vi "数值运算讲解.vi"() -> ()   [LabVIEW 2018]
uses:
  <vilib>/express/express arith-compare/Formula/XNode/ExpressFormulaBlockNode.xnode
panel:
  out "结果 2":dbl
  in  "X2":dbl
  in  "a 2":dbl
  out "y1":dbl
  in  "x":dbl
  out "数值 2":dbl
  in  "数值":dbl
  out "y":dbl
  in  "b":dbl
  in  "a":dbl
  out "结果":dbl
  in  "值 3":dbl
  in  "值 2":dbl
  in  "值":dbl
  # "y=2*a+b^2+5"
  # "y=x^2+3"
  # "y=a^2+x1^3"
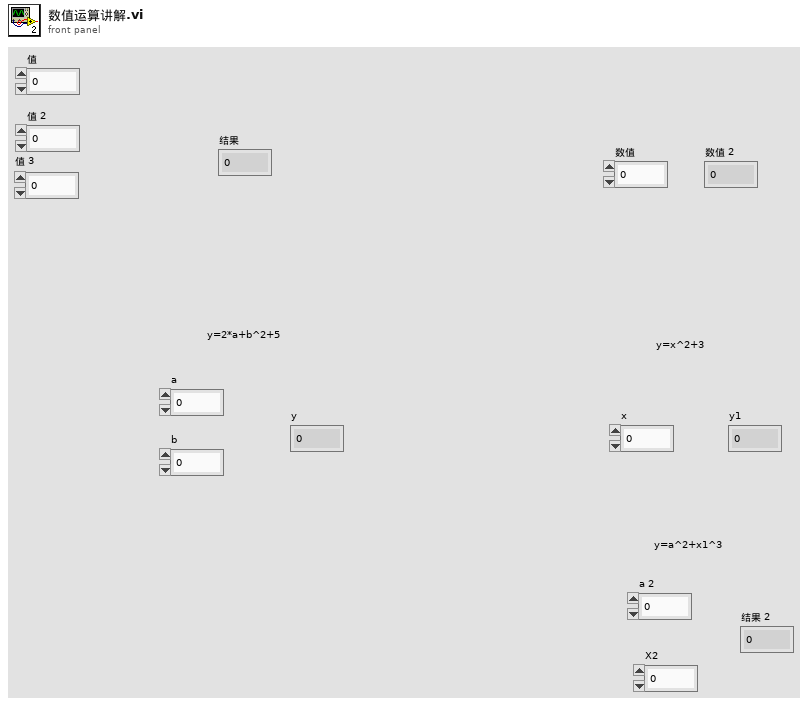
[diagram p1: front panel]
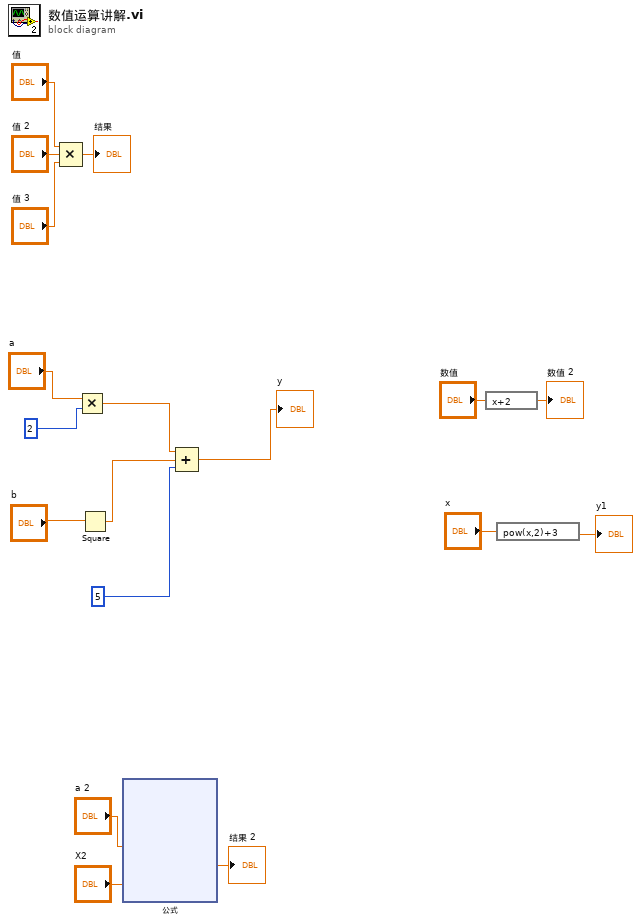
[diagram p0: block diagram]
diagram:
  n1 = Compound Arithmetic op=MULTIPLY("值", "值 2", "值 3") -> (→"结果":dbl)
  n2 = Multiply(x="a", y=2) -> (x*y=w9:dbl)
  n3 = Square(x="b") -> (x^2=w10:dbl)
  n4 = xnode "公式"("a"="a 2", "X2"="X2") -> ("结果"=→"结果 2":dbl)  [unwired: 1 in, 1 out]
  n5 = Compound Arithmetic op=ADD(w9, w10, 5) -> (→"y":dbl)
  n6 = expression code="x+2"("数值") -> (→"数值 2":dbl)
  n7 = expression code="pow(x,2)+3"("x") -> (→"y1":dbl)
